vi "Get RPC Service Name from Method Namespace.vi"(1 "RPC Method Name":string) -> (0 "RPC Service Name":string)   [LabVIEW 2019, in "gRPC Template Creation Utility.lvlib"]
uses:
  gRPC Template Creation Utility.lvlib
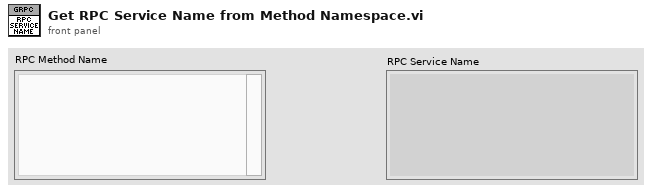
[diagram p1: front panel]
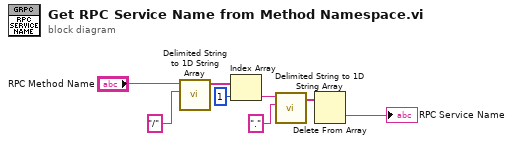
[diagram p0: block diagram]
diagram:
  n1 = call <vilib>:"Delimited String to 1D String Array.vi"("delimiter"="/", "delimited string"="RPC Method Name") -> ("string array"=w7:string[])  [unwired: 9 in]
  n2 = Index Array(array=w7, index=1) -> (element=w5:string)
  n3 = call <vilib>:"Delimited String to 1D String Array.vi"("delimiter"=".", "delimited string"=w5) -> ("string array"=w3:string[])  [unwired: 9 in]
  n4 = Delete From Array(array=w3) -> (deleted portion=→"RPC Service Name":string)  [unwired: 2 in, 1 out]
